vi "Wait on Server Loop.vi"(8 "error in (no error)":errorcluster, 10 "Value":bool, 11 "Websocket Server in":refnum<class "Websocket Server.lvclass">) -> (0 "error out":errorcluster, 3 "Websocket Server out":refnum<class "Websocket Server.lvclass">)   [LabVIEW 2020, in "Stream-Websocket.lvlib" / "Websocket Server.lvclass"]
uses:
  Websocket Server.lvclass
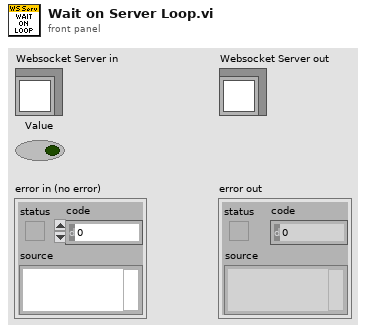
[diagram p1: front panel]
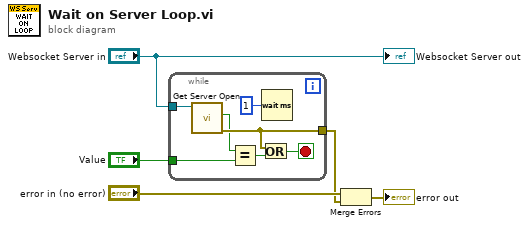
[diagram p0: block diagram]
diagram:
  n1 = while {
    tunnel: "Websocket Server in" -> [w12]
    tunnel: [w11] -> w1
    tunnel: "Value" -> [w7]
    stop <- w10 stop-if-true
    n2 = call "Get Server Open.vi"("Websocket Server in"=w12) -> ("error out"=w11:errorcluster, "Server Open"=w8:bool)  [unwired: 8 in, 1 out]
    n3 = Equal?(x=w8, y=w7) -> (x = y?=w9:bool)
    n4 = Or(x=w11, y=w9) -> (x .or. y?=w10:bool)
    n5 = Wait (ms)(milliseconds to wait=u32 1) -> ()  [unwired: 1 out]
  }
  n6 = Merge Errors("error in (no error)", w1) -> (→"error out":errorcluster)
  "Websocket Server out" <- "Websocket Server in"
